vi "Autonomous Independent.vi"   [LabVIEW 2014]
doc: "This VI is called when autonomous begins, and will automatically be terminated when autonomous ends. You can carry out timed or sensor driven robot movement independently without needing to return to the caller."
uses:
  <vilib>/Rock Robotics/WPI/Solenoid/WPI_SolenoidValue.ctl
  <vilib>/Rock Robotics/Network Tables/SD Read Number.vi
  Global Variables.vi
  <vilib>/Rock Robotics/WPI/Solenoid/WPI_SolenoidSetEnum.vi
types:
  T1 = typedef "WPI_SolenoidValue.ctl" = enum16{"Off", "On", "Forward", "Reverse"}
  T2 = typedef "WPI_MotorControlDeviceRef.ctl" = cluster{"DeviceStatus":errorcluster, "Type":T3, "PWM":cluster{"Controller":T4, "PWM Channel":T5, "DeadBand":T6}, "CAN":cluster{"Device Number":u8, "Control Mode":T7, "Semaphore":T8, "Max Vout":dbl, "TalonSRX Control Mode":T9}, "Invert":bool, "TransformRef":T10, "InvTransformRef":T10}
  T3 = typedef "WPI_MotorControlType.ctl" = enum16{"PWM", "CAN", "CANTalonSRX"}
  T4 = typedef "FPGA_TypedefDigitalModule.ctl" = enum16{"Controller 1"}
  T5 = typedef "FPGA_DIOPWMChannel.ctl" = enum8{"PWM 0", "PWM 1", "PWM 2", "PWM 3", "PWM 4", "PWM 5", "PWM 6", "PWM 7", "PWM 8", "PWM 9", "PWM MXP 0", "PWM MXP 1", "PWM MXP 2", "PWM MXP 3", "PWM MXP 4", "PWM MXP 5", "PWM MXP 6", "PWM MXP 7", "PWM MXP 8", "PWM MXP 9", "Invalid"}
  T6 = typedef "WPI_PWMDeadband.ctl" = cluster{"Name":string, "maxPositivePwm":i32, "minPositivePwm":i32, "centerPwm":i32, "maxNegativePwm":i32, "minNegativePwm":i32, "angularRange":u16}
  T7 = typedef "WPI_CANJaguar_ControlMode.ctl" = enum8{"Percent VBus", "Current", "Speed", "Position", "Voltage"}
  T8 = typedef "Semaphore RefNum" = refnum<k1>
  T9 = typedef "WPI_CANTalonSRX_APIControlMode.ctl" = enum8{"Percent VBus", "Speed", "Position", "Slave", "Unchanged / Invalid"}
  T10 = typedef "WPI_PWMTransform_ConPane.ctl" = refnum<vi>
  T11 = typedef "WPI_GyroDevRef.ctl" = cluster{"DevStatus":errorcluster, "Analog Module":T12, "Analog Channel":T13, "Offset":dbl, "Gain (VoltsPerDegree/Second)":dbl}
  T12 = typedef "FPGA_TypedefAnalogModule.ctl" = enum16{"Controller 1"}
  T13 = typedef "FPGA_AIChannel.ctl" = enum8{"AI 0", "AI 1", "AI 2", "AI 3", "AI MXP 0", "AI MXP 1", "AI MXP 2", "AI MXP 3", "Invalid"}
  T14 = typedef "WPI_SolenoidDevRef.ctl" = cluster{"DevStatus":errorcluster, "Pneumatics Control Module":u8, "Forward Solenoid Channel":T15, "Reverse Solenoid Channel":T15}
  T15 = typedef "WPI_SolenoidChannel.ctl" = enum8{"Solenoid 0", "Solenoid 1", "Solenoid 2", "Solenoid 3", "Solenoid 4", "Solenoid 5", "Solenoid 6", "Solenoid 7", "Invalid"}
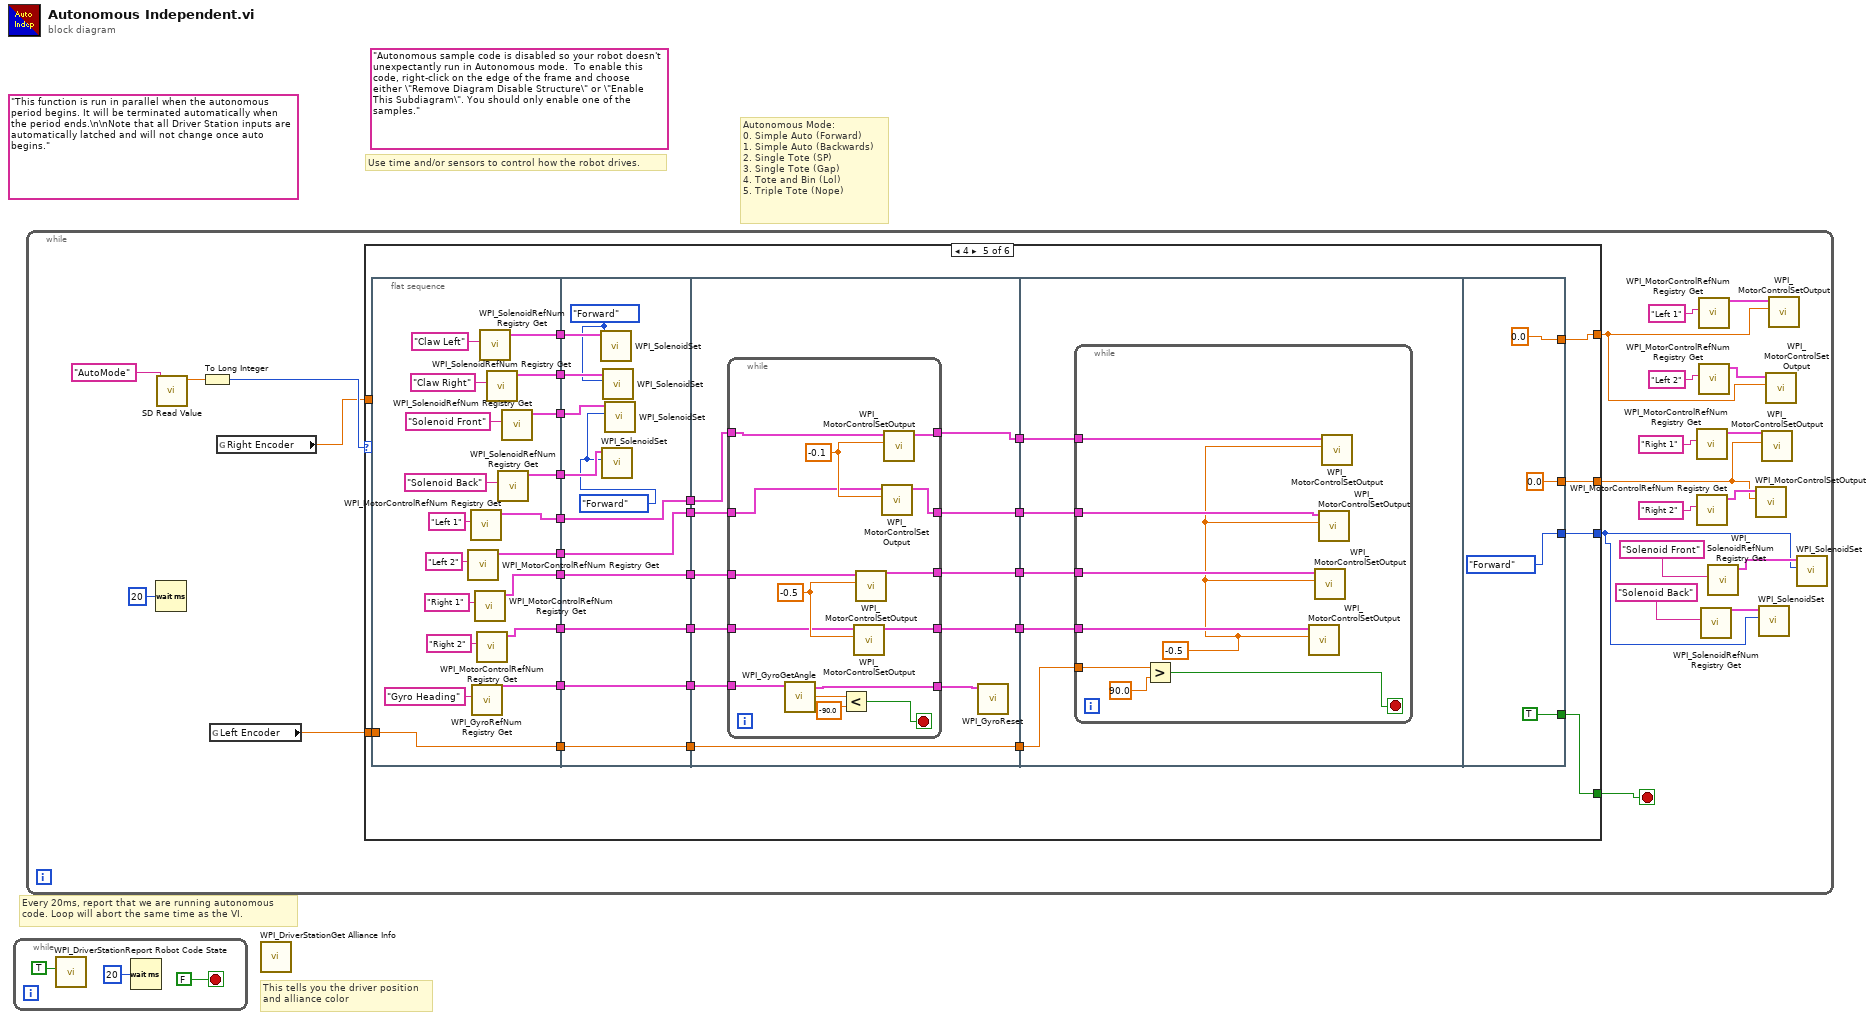
[diagram p0: block diagram]
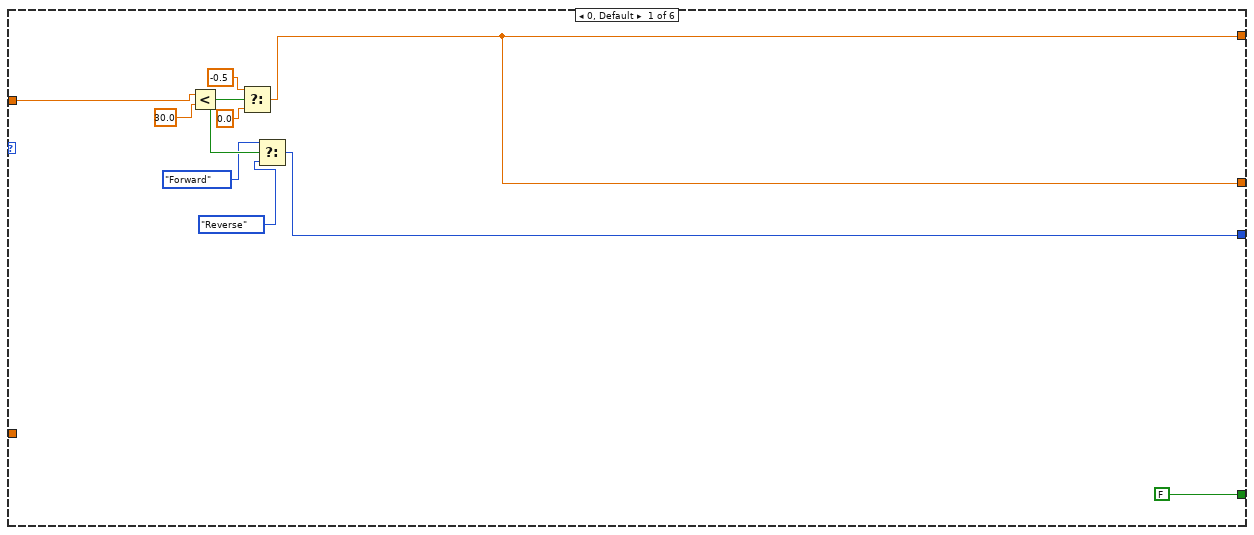
[diagram p2: hidden frame]
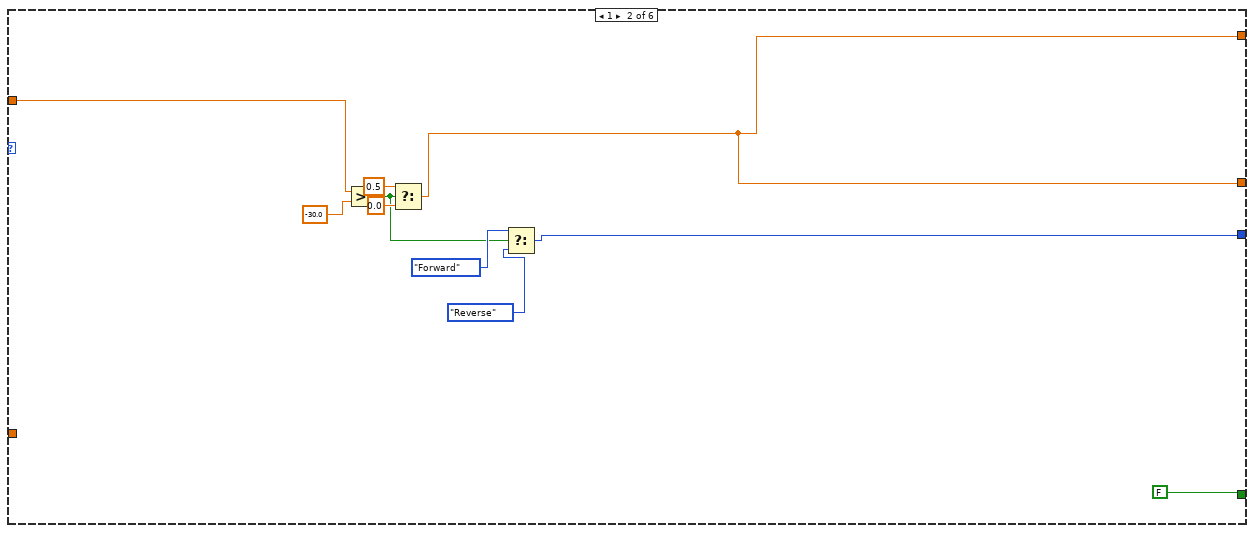
[diagram p3: hidden frame]
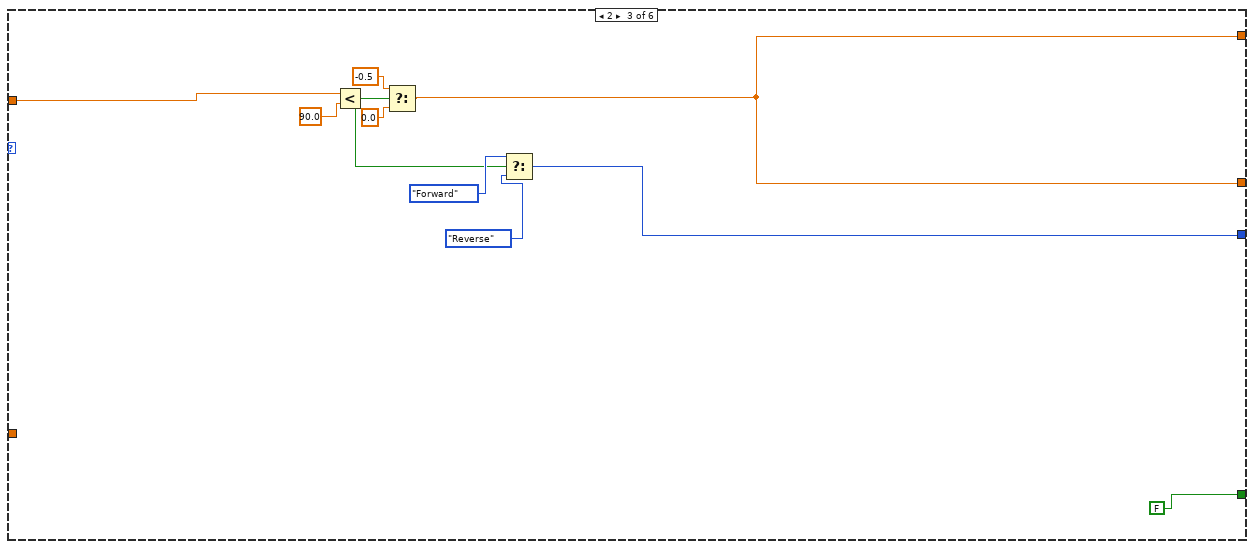
[diagram p4: hidden frame]
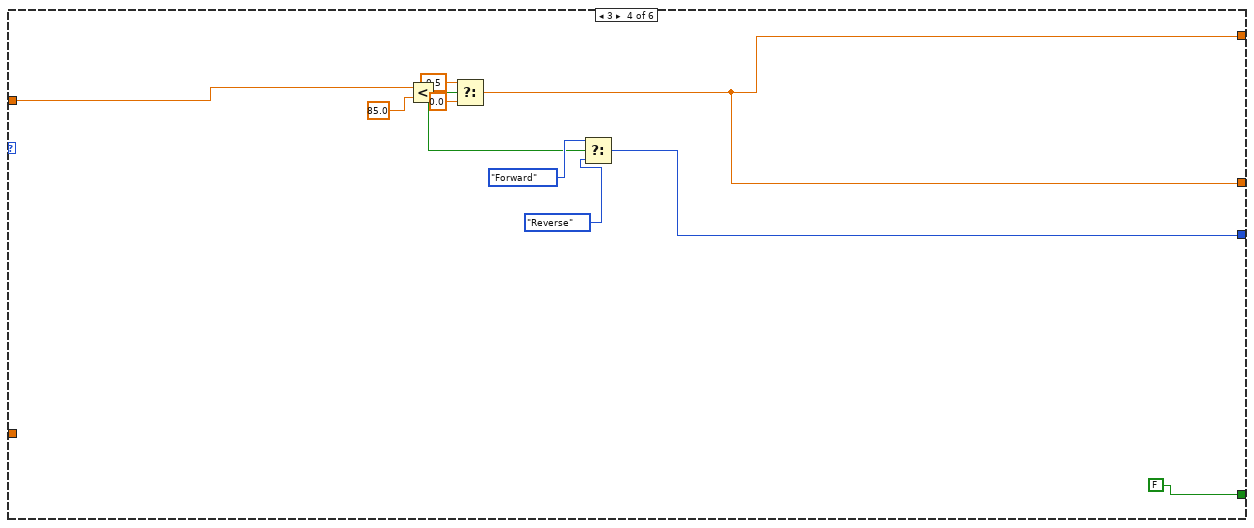
[diagram p5: hidden frame]
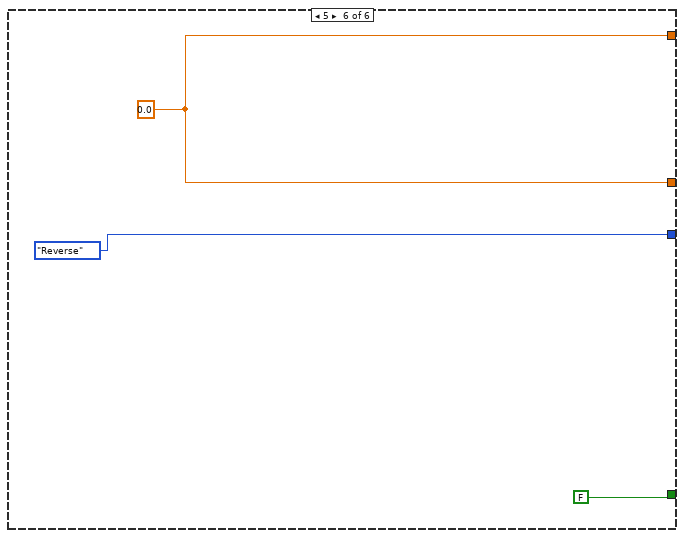
[diagram p6: hidden frame]
diagram:
  (unwired) "Autonomous sample code is disabled so your robot doesn't unexpectantly run in Autonomous mode.  To enable this code, right-click on the edge of the frame and choose either \"Remove Diagram Disable Structure\" or \"Enable This Subdiagram\". You should only enable one of the samples."
  (unwired) "This function is run in parallel when the autonomous period begins. It will be terminated automatically when the period ends.\n\nNote that all Driver Station inputs are automatically latched and will not change once auto begins."
  # "Autonomous Mode:\n0. Simple Auto (Forward)\n1. Simple Auto (Backwards)\n2. Single Tote (SP)\n3. Single Tote (Gap)\n4. Tote and Bin (Lol)\n5. Triple Tote (Nope)"
  # "Every 20ms, report that we are running autonomous\ncode. Loop will abort the same time as the VI."
  # "Use time and/or sensors to control how the robot drives."
  # "This tells you the driver position\nand alliance color"
  n1 = while {
    stop <- FALSE stop-if-true
    n2 = call <vilib>:"WPI_DriverStationReport Robot Code State.vi"("Autonomous"=TRUE) -> ()  [unwired: 10 in, 1 out]
    n3 = Wait (ms)(milliseconds to wait=u32 20) -> ()  [unwired: 1 out]
  }
  n4 = while {
    stop <- w5 stop-if-true
    n5 = Wait (ms)(milliseconds to wait=u32 20) -> ()  [unwired: 1 out]
    n6 = call-poly <vilib>:"SD Read Value.vi"("Name"="AutoMode") -> ("Numeric"=w24:dbl)  [unwired: 8 in, 2 out]
    n7 = To Long Integer(number=w24) -> (32bit integer=w23:i32)
    n8 = global read "Global Variables.vi" "Left Encoder"() -> (w4:dbl)
    n9 = global read "Global Variables.vi" "Right Encoder"() -> (w12:dbl)
    n10 = case shown="4" w23 {
      tunnel: [w33 w43 w53 w62 w66 w168] -> w15
      tunnel: [w33 w43 w53 w62 w67 w168] -> w14
      tunnel: w12 -> [w31 w41 w51 w61 _ _]
      tunnel: [w27 w37 w48 w58 w68 WPI_SolenoidValue."Reverse" ("Value")] -> w6
      tunnel: [FALSE FALSE FALSE FALSE w69 FALSE] -> w5
      tunnel: w4 -> [_ _ _ _ w70 _]
      frame 0, Default {
        n11 = Less?(x=w31, y=30.0) -> (x < y?=w30:bool)
        n12 = Select(t=-0.5, s=w30, f=0.0) -> (s? t:f=w33:dbl)
        n13 = Select(t=WPI_SolenoidValue."Forward" ("Value"), s=w30, f=WPI_SolenoidValue."Reverse" ("Value")) -> (s? t:f=w27:T1)
      }
      frame 1 {
        n14 = Greater?(x=w41, y=-30.0) -> (0:w38:bool)
        n15 = Select(t=0.5, s=w38, f=0.0) -> (s? t:f=w43:dbl)
        n16 = Select(t=WPI_SolenoidValue."Forward" ("Value"), s=w38, f=WPI_SolenoidValue."Reverse" ("Value")) -> (s? t:f=w37:T1)
      }
      frame 2 {
        n17 = Less?(x=w51, y=90.0) -> (x < y?=w47:bool)
        n18 = Select(t=-0.5, s=w47, f=0.0) -> (s? t:f=w53:dbl)
        n19 = Select(t=WPI_SolenoidValue."Forward" ("Value"), s=w47, f=WPI_SolenoidValue."Reverse" ("Value")) -> (s? t:f=w48:T1)
      }
      frame 3 {
        n20 = Less?(x=w61, y=85.0) -> (x < y?=w57:bool)
        n21 = Select(t=-0.5, s=w57, f=0.0) -> (s? t:f=w62:dbl)
        n22 = Select(t=WPI_SolenoidValue."Forward" ("Value"), s=w57, f=WPI_SolenoidValue."Reverse" ("Value")) -> (s? t:f=w58:T1)
      }
      frame 4 {
        n23 = flat-sequence {
          tunnel: [w101] -> w91
          tunnel: [w100] -> w90
          tunnel: [w99] -> w89
          tunnel: [w98] -> w88
          tunnel: [w97] -> w87
          tunnel: [w96] -> w85
          tunnel: [w95] -> w82
          tunnel: [w94] -> w77
          tunnel: [w93] -> w76
          tunnel: [w92] -> w71
          tunnel: w70 -> [w92]
          tunnel: w91 -> [w122]
          tunnel: w90 -> [w121]
          tunnel: w89 -> [w120]
          tunnel: w88 -> [w119]
          tunnel: w87 -> [w116]
          tunnel: [w116] -> w86
          tunnel: w85 -> [w115]
          tunnel: [w115] -> w84
          tunnel: [w114] -> w83
          tunnel: w82 -> [w114]
          tunnel: [w113] -> w78
          tunnel: w77 -> [w113]
          tunnel: w76 -> [w112]
          tunnel: [w112] -> w75
          tunnel: [w111] -> w72
          tunnel: w71 -> [w111]
          tunnel: w86 -> [w133]
          tunnel: w84 -> [w132]
          tunnel: w83 -> [w131]
          tunnel: [w129] -> w81
          tunnel: [w128] -> w80
          tunnel: [w124] -> w79
          tunnel: w78 -> [w123]
          tunnel: w75 -> [w125]
          tunnel: [w126] -> w74
          tunnel: [w127] -> w73
          tunnel: w72 -> [w127]
          tunnel: w81 -> [w153]
          tunnel: w80 -> [w152]
          tunnel: w79 -> [w151]
          tunnel: w74 -> [w150]
          tunnel: w73 -> [w149]
          tunnel: [TRUE] -> w69
          tunnel: [WPI_SolenoidValue."Forward" ("Value")] -> w68
          tunnel: [0.0] -> w67
          tunnel: [0.0] -> w66
          frame #0 {
            n24 = call <vilib>:"WPI_MotorControlRefNum Registry Get.vi"("refnum name"="Left 2") -> ("MotorControlDevRef"=w94:T2)  [unwired: 9 in, 1 out]
            n25 = call <vilib>:"WPI_MotorControlRefNum Registry Get.vi"("refnum name"="Left 1") -> ("MotorControlDevRef"=w93:T2)  [unwired: 9 in, 1 out]
            n26 = call <vilib>:"WPI_GyroRefNum Registry Get.vi"("refnum name"="Gyro Heading") -> ("GyroDevRef"=w97:T11)  [unwired: 9 in, 1 out]
            n27 = call <vilib>:"WPI_MotorControlRefNum Registry Get.vi"("refnum name"="Right 1") -> ("MotorControlDevRef"=w95:T2)  [unwired: 9 in, 1 out]
            n28 = call <vilib>:"WPI_MotorControlRefNum Registry Get.vi"("refnum name"="Right 2") -> ("MotorControlDevRef"=w96:T2)  [unwired: 9 in, 1 out]
            n29 = call <vilib>:"WPI_SolenoidRefNum Registry Get.vi"("refnum name"="Claw Left") -> ("SolenoidDevRef"=w98:T14)  [unwired: 9 in, 1 out]
            n30 = call <vilib>:"WPI_SolenoidRefNum Registry Get.vi"("refnum name"="Claw Right") -> ("SolenoidDevRef"=w99:T14)  [unwired: 9 in, 1 out]
            n31 = call <vilib>:"WPI_SolenoidRefNum Registry Get.vi"("refnum name"="Solenoid Back") -> ("SolenoidDevRef"=w101:T14)  [unwired: 9 in, 1 out]
            n32 = call <vilib>:"WPI_SolenoidRefNum Registry Get.vi"("refnum name"="Solenoid Front") -> ("SolenoidDevRef"=w100:T14)  [unwired: 9 in, 1 out]
          }
          frame #1 {
            w117 = WPI_SolenoidValue."Forward" ("Value")
            w118 = WPI_SolenoidValue."Forward" ("Value")
            n33 = call-poly <vilib>:"WPI_SolenoidSet.vi"("Value"=w118, "SolenoidDevRef"=w119) -> ()  [unwired: 8 in, 2 out]
            n34 = call-poly <vilib>:"WPI_SolenoidSet.vi"("Value"=w117, "SolenoidDevRef"=w122) -> ()  [unwired: 8 in, 2 out]
            n35 = call-poly <vilib>:"WPI_SolenoidSet.vi"("Value"=w118, "SolenoidDevRef"=w120) -> ()  [unwired: 8 in, 2 out]
            n36 = call-poly <vilib>:"WPI_SolenoidSet.vi"("Value"=w117, "SolenoidDevRef"=w121) -> ()  [unwired: 8 in, 2 out]
          }
          frame #2 {
            n37 = while {
              tunnel: w133 -> [w148]
              tunnel: w132 -> [w143]
              tunnel: w131 -> [w142]
              tunnel: [w141] -> w130
              tunnel: [w140] -> w129
              tunnel: [w139] -> w128
              tunnel: [w137] -> w126
              tunnel: w125 -> [w134]
              tunnel: [w136] -> w124
              tunnel: w123 -> [w135]
              stop <- w145 stop-if-true
              w138 = -0.1
              w144 = -0.5
              n38 = call <vilib>:"WPI_GyroGetAngle.vi"("GyroDevRef"=w148) -> ("Angle"=w147:dbl, "GyroDevRef"=w141:T11)  [unwired: 7 in, 2 out]
              n39 = Less?(x=w147, y=-90.0) -> (x < y?=w145:bool)
              n40 = call <vilib>:"WPI_MotorControlSetOutput.vi"("Output"=w144, "MotorControlDevRef"=w143) -> ("MotorControlDevRef"=w140:T2)  [unwired: 7 in, 2 out]
              n41 = call <vilib>:"WPI_MotorControlSetOutput.vi"("Output"=w144, "MotorControlDevRef"=w142) -> ("MotorControlDevRef"=w139:T2)  [unwired: 7 in, 2 out]
              n42 = call <vilib>:"WPI_MotorControlSetOutput.vi"("Output"=w138, "MotorControlDevRef"=w135) -> ("MotorControlDevRef"=w136:T2)  [unwired: 7 in, 2 out]
              n43 = call <vilib>:"WPI_MotorControlSetOutput.vi"("Output"=w138, "MotorControlDevRef"=w134) -> ("MotorControlDevRef"=w137:T2)  [unwired: 7 in, 2 out]
            }
            n44 = call <vilib>:"WPI_GyroReset.vi"("GyroDevRef"=w130) -> ()  [unwired: 9 in, 2 out]
          }
          frame #3 {
            n45 = while {
              tunnel: w153 -> [w161]
              tunnel: w152 -> [w160]
              tunnel: w151 -> [w159]
              tunnel: w150 -> [w158]
              tunnel: w149 -> [w156]
              stop <- w154 stop-if-true
              w155 = -0.5 ("t")
              n46 = Greater?(x=w156, y=90.0) -> (0:w154:bool)
              n47 = call <vilib>:"WPI_MotorControlSetOutput.vi"("Output"=w155, "MotorControlDevRef"=w161) -> ()  [unwired: 7 in, 3 out]
              n48 = call <vilib>:"WPI_MotorControlSetOutput.vi"("Output"=w155, "MotorControlDevRef"=w160) -> ()  [unwired: 7 in, 3 out]
              n49 = call <vilib>:"WPI_MotorControlSetOutput.vi"("Output"=w155, "MotorControlDevRef"=w159) -> ()  [unwired: 7 in, 3 out]
              n50 = call <vilib>:"WPI_MotorControlSetOutput.vi"("Output"=w155, "MotorControlDevRef"=w158) -> ()  [unwired: 7 in, 3 out]
            }
          }
          frame #4 {
          }
        }
      }
      frame 5 {
        w168 = 0.0
      }
    }
    n51 = call <vilib>:"WPI_MotorControlRefNum Registry Get.vi"("refnum name"="Right 1") -> ("MotorControlDevRef"=w17:T2)  [unwired: 9 in, 1 out]
    n52 = call <vilib>:"WPI_MotorControlRefNum Registry Get.vi"("refnum name"="Right 2") -> ("MotorControlDevRef"=w16:T2)  [unwired: 9 in, 1 out]
    n53 = call <vilib>:"WPI_MotorControlRefNum Registry Get.vi"("refnum name"="Left 1") -> ("MotorControlDevRef"=w18:T2)  [unwired: 9 in, 1 out]
    n54 = call <vilib>:"WPI_MotorControlRefNum Registry Get.vi"("refnum name"="Left 2") -> ("MotorControlDevRef"=w19:T2)  [unwired: 9 in, 1 out]
    n55 = call <vilib>:"WPI_SolenoidRefNum Registry Get.vi"("refnum name"="Solenoid Back") -> ("SolenoidDevRef"=w7:T14)  [unwired: 9 in, 1 out]
    n56 = call <vilib>:"WPI_SolenoidRefNum Registry Get.vi"("refnum name"="Solenoid Front") -> ("SolenoidDevRef"=w8:T14)  [unwired: 9 in, 1 out]
    n57 = call <vilib>:"WPI_MotorControlSetOutput.vi"("Output"=w14, "MotorControlDevRef"=w16) -> ()  [unwired: 7 in, 3 out]
    n58 = call-poly <vilib>:"WPI_SolenoidSet.vi"("Value"=w6, "SolenoidDevRef"=w7) -> ()  [unwired: 8 in, 2 out]
    n59 = call <vilib>:"WPI_MotorControlSetOutput.vi"("Output"=w14, "MotorControlDevRef"=w17) -> ()  [unwired: 7 in, 3 out]
    n60 = call <vilib>:"WPI_MotorControlSetOutput.vi"("Output"=w15, "MotorControlDevRef"=w19) -> ()  [unwired: 7 in, 3 out]
    n61 = call <vilib>:"WPI_MotorControlSetOutput.vi"("Output"=w15, "MotorControlDevRef"=w18) -> ()  [unwired: 7 in, 3 out]
    n62 = call-poly <vilib>:"WPI_SolenoidSet.vi"("Value"=w6, "SolenoidDevRef"=w8) -> ()  [unwired: 8 in, 2 out]
  }
  n63 = call <vilib>:"WPI_DriverStationGet Alliance Info.vi"() -> ()  [unwired: 12 out]
